vi "Compute DistanceToTarget.vi"(8 "Y Image Resolution":i32=240, 9 "X Image Resolution":i32=320, 10 "Vertical Strip":T1={"Horizontal"=FALSE, "Aspect Score"=62.73913077154114, "Rect Score"=78.14814814814815, "Rectangle"={"Left"=165.0, "Top"=109.0, "Right"=170.0, "Bottom"=163.0}, "Equiv H"=4.067855176993643, "Equiv V"=51.87008652455029}, 11 "Camera Type":enum16{"206", "1011", "1013"}(ring)=enum."1011") -> (2 "Target Center (-1 to 1)":cluster{"X":dbl, "Y":dbl}={"X"=0.046875, "Y"=0.13333333333333333}, 3 "Distance (ft)":dbl=18.43797171275333)   [LabVIEW 2013]
doc: "Using the camera lens information and the real world size of the target, use trig and ratios to determine the distance to the target. Also returns the location relative to the image center in a (-1 , 1) coordinate system that may be useful for steering the robot."
panel:
  in  "Camera view angles":dbl[](array[numeric])=[41.7, 37.0, 49.0]
  # "Axis 206\nAxis M1011\nAxis M1013"
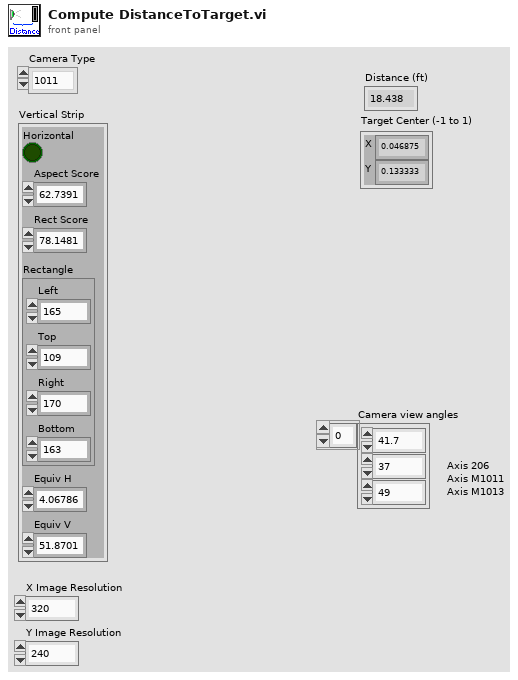
[diagram p1: front panel]
types:
  T1 = cluster{"Horizontal":bool, "Aspect Score":dbl, "Rect Score":dbl, "Rectangle":cluster{"Left":dbl, "Top":dbl, "Right":dbl, "Bottom":dbl}, "Equiv H":dbl, "Equiv V":dbl}
  T2 = cluster{"X Image Resolution":i32, "Y Image Resolution":i32}
  T3 = cluster{"X Image Resolution":dbl, "Y Image Resolution":dbl}
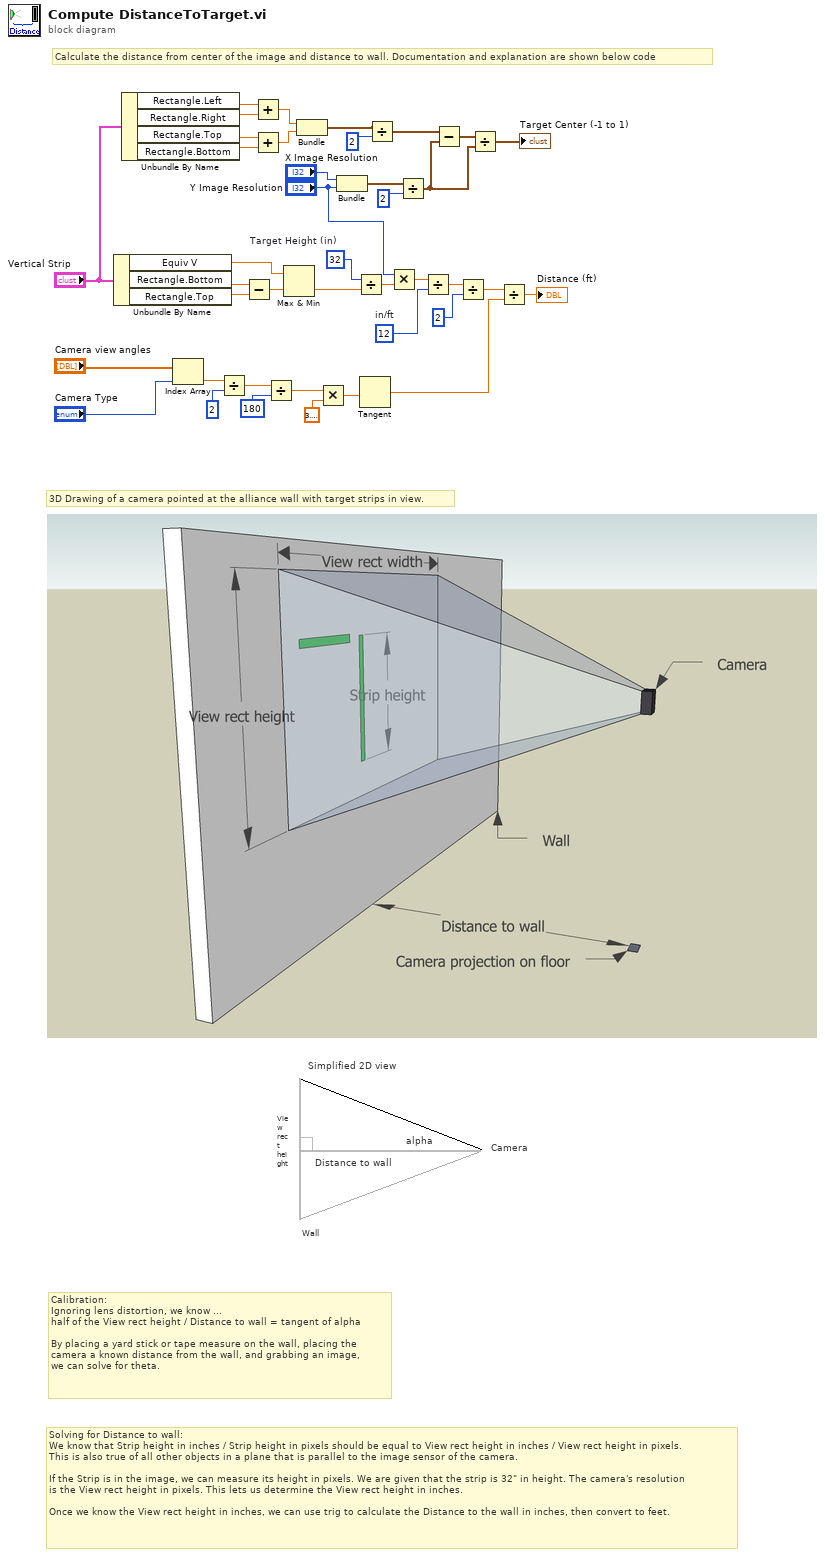
[diagram p0: block diagram]
diagram:
  w6 = 12  # in/ft
  w11 = 32  # Target Height (in)
  # "Wall"
  # "Camera"
  # "Simplified 2D view"
  # "Solving for Distance to wall:\nWe know that Strip height in inches / Strip height in pixels should be equal to View rect height in inches / View rect height in pixels.\nThis is also true of all other objects in a plane that is parallel to the image sensor of the camera.\n\nIf the Strip is in the image, we can measure its height in pixels. We are given that the strip is 32\" in height. The camera's resolution\nis the View rect height in pixels. This lets us determine the View rect height in inches.\n\nOnce we know the View rect height in inches, we can use trig to calculate the Distance to the wall in inches, then convert to feet."
  # "3D Drawing of a camera pointed at the alliance wall with target strips in view."
  # "Distance to wall"
  # "View rect height"
  # "alpha"
  # "Calibration:\nIgnoring lens distortion, we know ...\nhalf of the View rect height / Distance to wall = tangent of alpha\n\nBy placing a yard stick or tape measure on the wall, placing the\ncamera a known distance from the wall, and grabbing an image,\nwe can solve for theta."
  # "Calculate the distance from center of the image and distance to wall. Documentation and explanation are shown below code"
  n1 = Unbundle By Name("Vertical Strip") -> ("Equiv V"=w14:dbl, "Rectangle.Bottom"=w31:dbl, "Rectangle.Top"=w30:dbl)
  n2 = Unbundle By Name("Vertical Strip") -> ("Rectangle.Left"=w25:dbl, "Rectangle.Right"=w26:dbl, "Rectangle.Top"=w28:dbl, "Rectangle.Bottom"=w27:dbl)
  n3 = Index Array(array="Camera view angles", index="Camera Type") -> (element=w37:dbl)
  n4 = Divide(x=w37, y=2) -> (x/y=w34:dbl)
  n5 = Subtract(x=w31, y=w30) -> (x-y=w13:dbl)
  n6 = Add(x=w25, y=w26) -> (x+y=w23:dbl)
  n7 = Add(x=w28, y=w27) -> (x+y=w22:dbl)
  n8 = Divide(x=w34, y=180) -> (x/y=w33:dbl)
  n9 = Max & Min(x=w14, y=w13) -> (min(x,y)=w10:dbl)  [unwired: 1 out]
  n10 = Bundle(w23, w22) -> (w19:cluster{dbl, dbl})  [unwired: 1 in]
  n11 = Multiply(x=w33, y=3.141592653589793) -> (x*y=w35:dbl)
  n12 = Bundle("X Image Resolution"="X Image Resolution", "Y Image Resolution"="Y Image Resolution") -> (w21:T2)  [unwired: 1 in]
  n13 = Divide(x=w11, y=w10) -> (x/y=w9:dbl)
  n14 = Tangent(1:w35) -> (0:w2:dbl)
  n15 = Divide(x=w19, y=2) -> (x/y=w18:cluster{dbl, dbl})
  n16 = Multiply(x="Y Image Resolution", y=w9) -> (x*y=w7:dbl)
  n17 = Divide(x=w21, y=2) -> (x/y=w16:T3)
  n18 = Divide(x=w7, y=w6) -> (x/y=w5:dbl)
  n19 = Subtract(x=w18, y=w16) -> (x-y=w17:cluster{dbl, dbl})
  n20 = Divide(x=w5, y=2) -> (x/y=w3:dbl)
  n21 = Divide(x=w17, y=w16) -> (x/y=→"Target Center (-1 to 1)":cluster{dbl, dbl})
  n22 = Divide(x=w3, y=w2) -> (x/y=→"Distance (ft)":dbl)
